vi "red_tweezers_UNDO.vi"(5 "Force Save":bool, 7 "This change is inconsequential (don't save it)":bool, 8 "Selection/Group":T1[](array[typedef]), 10 "Undo/Store (store, False)":bool, 11 "Spots":T2[](array[typedef]) {"Amplitude Correction" step=0.1; "Line Trapping"."Phase Gradient" step=0.05; "Line Trapping"."Vector"."x" step=1e-06 format="%#_6p"; "Line Trapping"."Vector"."y" step=1e-06 format="%#_6p"; "Line Trapping"."Vector"."z" step=1e-06 format="%#_6p"; "NA Position"."r" step=1e-06; "NA Position"."y" step=1e-06; "NA Position"."x" step=1e-06; "Position"."z" step=1e-06; "Position"."y" step=1e-06; "Position"."x" step=1e-06; "Phase" step=0.7753; "Intensity" step=0.1}) -> (0 "Selection/Group Out (Undo only)":T1[](array[typedef]), 3 "Spots Out (Undo only)":T2[](array[typedef]) {"Amplitude Correction" step=0.1; "Line Trapping"."Phase Gradient" step=0.05; "Line Trapping"."Vector"."x" step=1e-06 format="%#_6p"; "Line Trapping"."Vector"."y" step=1e-06 format="%#_6p"; "Line Trapping"."Vector"."z" step=1e-06 format="%#_6p"; "NA Position"."r" step=1e-06; "NA Position"."y" step=1e-06; "NA Position"."x" step=1e-06; "Position"."z" step=1e-06; "Position"."y" step=1e-06; "Position"."x" step=1e-06; "Phase" step=0.7753; "Intensity" step=0.1})   [LabVIEW 2010]
doc: "The \"undo\" stack is maintained by this VI. By default, it saves an undo point each time what is wired into it changes. However, this can be altered with \"inconsequential\" (which stops changes being saved) and \"force\" (which makes sure it saves even if it's a duplicate).\n\nWhen it is called with \"Undo/Store\" true, it outputs the last undo point, and removes it from the list."
uses:
  selection_element.ctl
  spot.ctl
  line_trapping.ctl
panel:
  # "See context help on the boolean terminals for more details."
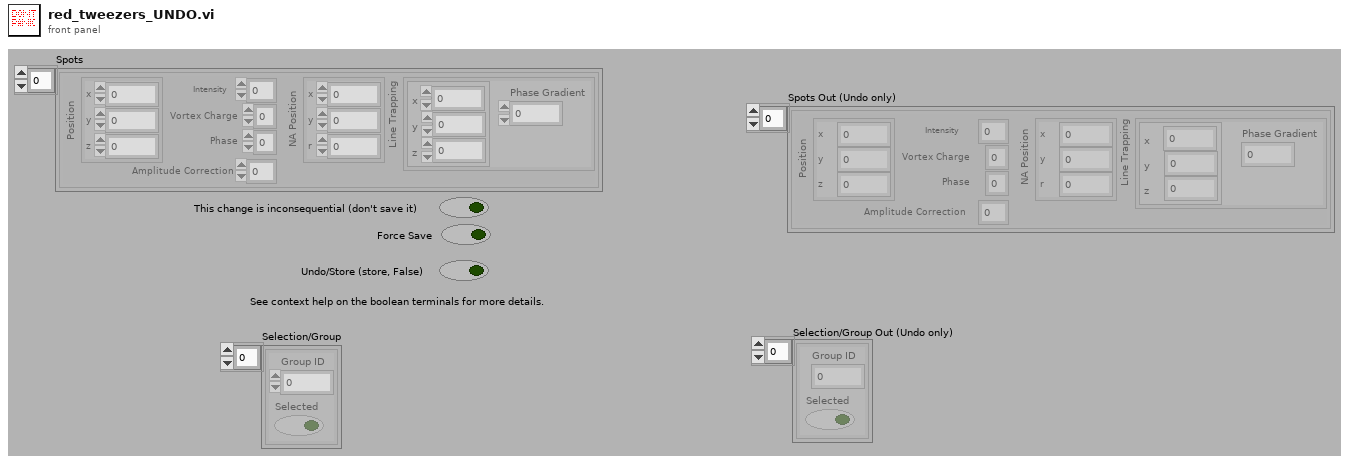
[diagram p1: front panel]
types:
  T1 = typedef "selection_element.ctl" = cluster{"Group ID":i32, "Selected":bool}
  T2 = typedef "spot.ctl" = cluster{"Position":cluster{"x":dbl, "y":dbl, "z":dbl}, "Intensity":dbl, "Vortex Charge":i8, "Phase":dbl, "NA Position":cluster{"x":dbl, "y":dbl, "r":dbl}, "Line Trapping":T3, "Amplitude Correction":dbl}
  T3 = typedef "line_trapping.ctl" = cluster{"Vector":cluster{"x":dbl, "y":dbl, "z":dbl}, "Phase Gradient":dbl}
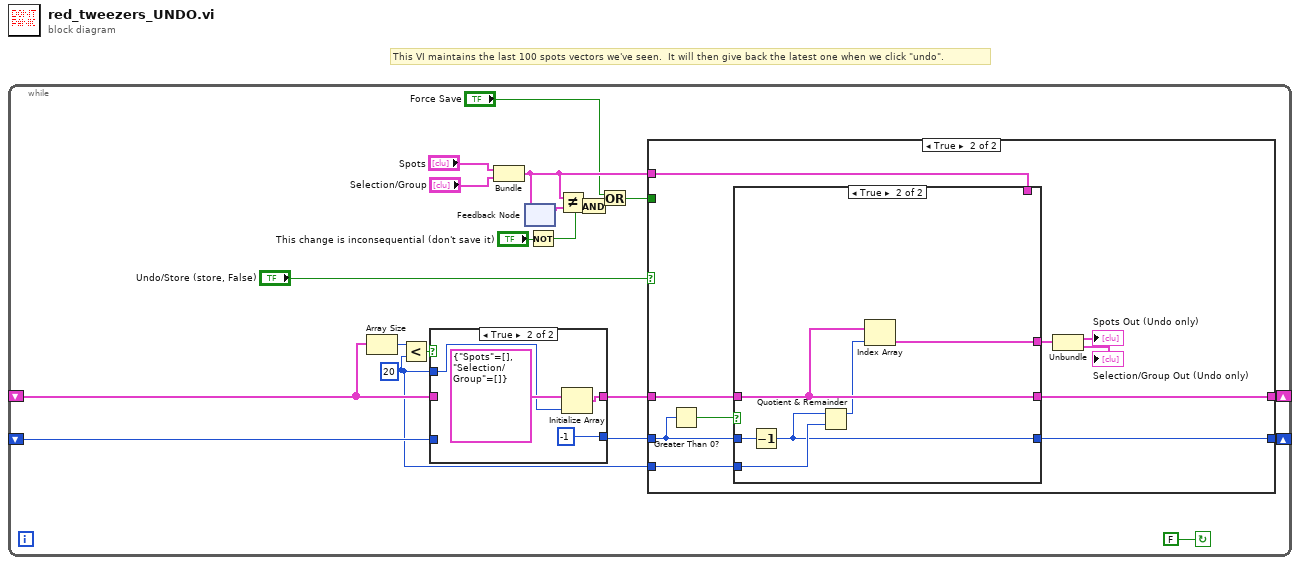
[diagram p0: block diagram]
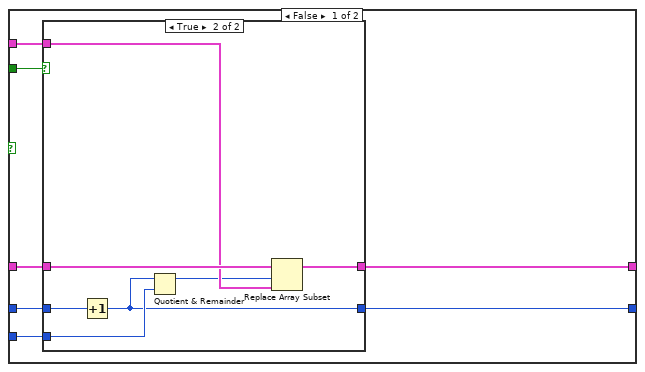
[diagram p2: hidden frame]
diagram:
  # "This VI maintains the last 100 spots vectors we've seen.  It will then give back the latest one when we click \"undo\"."
  n1 = while {
    shift-right: [w14] -> _
    shift-left: _ -> [w20]
    shift-right: [w13] -> _
    shift-left: _ -> [w17]
    stop <- FALSE continue-if-true
    w12 = 20 ("dimension size")
    n2 = Array Size(array=w20) -> (size(s)=w19:i32)
    n3 = Less?(x=w19, y=w12) -> (x < y?=w18:bool)
    n4 = case shown="True" w18 {
      tunnel: w12 -> [_ w61]
      tunnel: w20 -> [w58 _]
      tunnel: [w58 w60] -> w15
      tunnel: w17 -> [w57 _]
      tunnel: [w57 -1 ("dimension size")] -> w16
      frame False {
      }
      frame True {
        n5 = Initialize Array(cluster{"Spots":T2[], "Selection/Group":T1[]} {"Spots"=[], "Selection/Group"=[]} ("output cluster"), w61) -> (w60:cluster{"Spots":T2[], "Selection/Group":T1[]}[])
      }
    }
    n6 = Bundle("Spots"="Spots", "Selection/Group"="Selection/Group") -> (w11:cluster{"Spots":T2[], "Selection/Group":T1[]})  [unwired: 1 in]
    n7 = feedback #1() -> (w4:cluster{"Spots":T2[], "Selection/Group":T1[]})  [unwired: 1 in]
    n8 = feedback-in #1(w11) -> ()
    n9 = Not(x="This change is inconsequential (don't save it)") -> (.not. x?=w1:bool)
    n10 = Not Equal?(x=w11, y=w4) -> (x != y?=w8:bool)
    n11 = And(x=w8, y=w1) -> (x .and. y?=w3:bool)
    n12 = Or(x="Force Save", y=w3) -> (x .or. y?=w10:bool)
    n13 = case shown="True" "Undo/Store (store, False)" {
      tunnel: w16 -> [w27 w42]
      tunnel: w15 -> [w28 w46]
      tunnel: w11 -> [w26 w38]
      tunnel: [w25 w44] -> w14
      tunnel: [w23 w43] -> w13
      tunnel: w12 -> [w24 w45]
      tunnel: w10 -> [w22 _]
      frame False {
        n14 = case shown="True" w22 {
          tunnel: w28 -> [w30 w37]
          tunnel: w27 -> [w29 w36]
          tunnel: w26 -> [_ w35]
          tunnel: [w30 w34] -> w25
          tunnel: w24 -> [_ w32]
          tunnel: [w29 w31] -> w23
          frame False {
          }
          frame True {
            n15 = Increment(x=w36) -> (x+1=w31:i32)
            n16 = Quotient & Remainder(x=w31, y=w32) -> (x-y*floor(x/y)=w33:i32)  [unwired: 1 out]
            n17 = Replace Array Subset(array=w37, new element=w35, index=w33) -> (w34:cluster{"Spots":T2[], "Selection/Group":T1[]}[])
          }
        }
      }
      frame True {
        n18 = Greater Than 0?(x=w42) -> (x > 0?=w47:bool)
        n19 = case shown="True" w47 {
          tunnel: w46 -> [w49 w56]
          tunnel: w45 -> [_ w53]
          tunnel: [w49 w56] -> w44
          tunnel: [w48 w51] -> w43
          tunnel: w42 -> [w48 w52]
          tunnel: [w50 w55] -> w41
          tunnel: w38 -> [w50 _]
          frame False {
          }
          frame True {
            n20 = Decrement(x=w52) -> (x-1=w51:i32)
            n21 = Quotient & Remainder(x=w51, y=w53) -> (x-y*floor(x/y)=w54:i32)  [unwired: 1 out]
            n22 = Index Array(array=w56, index=w54) -> (element=w55:cluster{"Spots":T2[], "Selection/Group":T1[]})
          }
        }
        n23 = Unbundle(w41) -> ("Spots"=→"Spots Out (Undo only)":T2[], "Selection/Group"=→"Selection/Group Out (Undo only)":T1[])
      }
    }
  }
